vi "rohiteq.vi"() -> ()   [LabVIEW 2009]
panel:
  out "Numeric 3":dbl
  in  "Numeric 2":dbl
  in  "Numeric":dbl
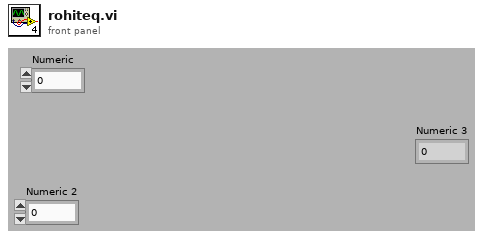
[diagram p1: front panel]
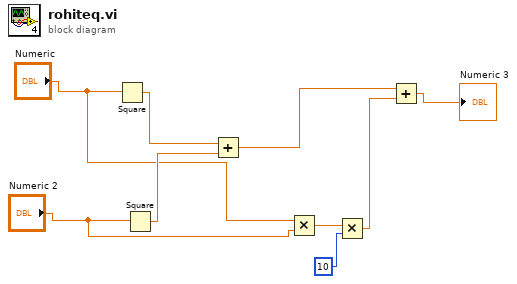
[diagram p0: block diagram]
diagram:
  n1 = Square(x="Numeric") -> (x^2=w9:dbl)
  n2 = Square(x="Numeric 2") -> (x^2=w8:dbl)
  n3 = Add(x=w9, y=w8) -> (x+y=w7:dbl)
  n4 = Multiply(x="Numeric", y="Numeric 2") -> (x*y=w4:dbl)
  n5 = Multiply(x=w4, y=10) -> (x*y=w2:dbl)
  n6 = Add(x=w7, y=w2) -> (x+y=→"Numeric 3":dbl)
